vi "ULx Read (Analog Wfm 1Chan NSamp).vi"(0 "task in":refnum<k24>, 7 "number of samples per channel":i32=-1, 9 "timeout":dbl=10.0 format="%_4g", 11 "error in":errorcluster) -> (4 "task out":refnum<k24>, 6 "data":waveform(dbl), 15 "error out":errorcluster)   [LabVIEW 2020]
doc: "Reads a waveform from a task that contains a single analog input channel."
uses:
  C:/Users/William/Documents/LV 2020 builds/LeaktestDAQ/Source-v33/ULx_LV.dll
  ULx_LV.dll
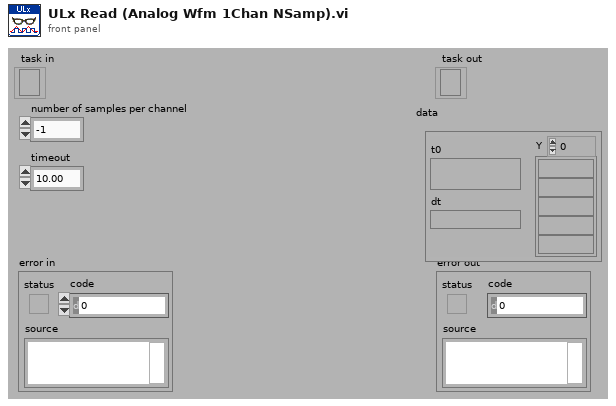
[diagram p1: front panel]
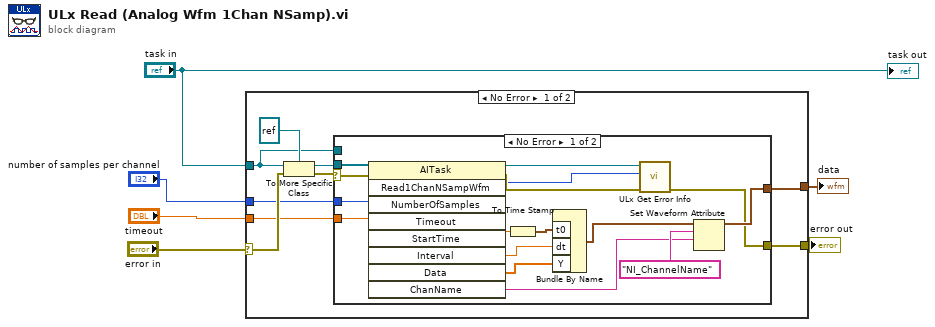
[diagram p0: block diagram]
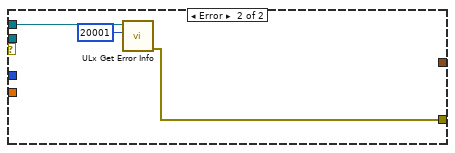
[diagram p2: hidden frame]
diagram:
  n1 = case shown="No Error" "error in" {
    selector: "error in" -> [w15 w35]
    tunnel: "task in" -> [w7 _]
    tunnel: "timeout" -> [w11 _]
    tunnel: [w8 _] -> w1
    tunnel: [w10 w35] -> w4
    tunnel: "number of samples per channel" -> [w9 _]
    frame No Error {
      n2 = To More Specific Class(target class=refnum<k24> refnum, reference=w7, error in=w15) -> (specific class reference=w12:refnum<k24>, error out=w13:errorcluster)
      n3 = case shown="No Error" w13 {
        selector: w13 -> [w30 _]
        tunnel: w12 -> [w31 _]
        tunnel: w11 -> [w28 _]
        tunnel: [w17 w32] -> w10
        tunnel: w9 -> [w27 _]
        tunnel: [w22 _] -> w8
        tunnel: w7 -> [_ w34]
        frame No Error {
          n4 = invoke class="AITask" method="Read1ChanNSampWfm"(reference=w31, error in=w30, "NumberOfSamples"=w27, "Timeout"=w28) -> (reference out=w29:refnum<k24>, error out=w18:errorcluster, "Read1ChanNSampWfm"=w16:i32, "StartTime"=w21:dbl, "Interval"=w20:dbl, "Data"=w19:dbl[], "ChanName"=w23:string)  [unwired: 5 in, 2 out]
          n5 = To Time Stamp(1:w21) -> (0:w26:timestamp)
          n6 = Bundle By Name("t0"=w26, "dt"=w20, "Y"=w19) -> (w25:waveform(dbl))  [unwired: 1 in]
          n7 = call "ULx Get Error Info.vi"("error in"=w18, "ErrorCode"=w16, "task in"=w29) -> ("error out"=w17:errorcluster)  [unwired: 8 in]
          n8 = Set Waveform Attribute(5:w23, 6:"NI_ChannelName", 7:w25) -> (3:w22:waveform(dbl))  [unwired: 1 in, 2 out]
        }
        frame Error {
          n9 = call "ULx Get Error Info.vi"("ErrorCode"=20001, "task in"=w34) -> ("error out"=w32:errorcluster)  [unwired: 9 in]
        }
      }
    }
    frame Error {
    }
  }
  "error out" <- w4
  "data" <- w1
  "task out" <- "task in"
